vi "DWF FGEN Query Waveform Mode.vi"(0 "Instrument Handle In":u32, 11 "Error In":errorcluster caption="Error In (no error)") -> (4 "Instrument Handle Out":u32, 6 "Waveform Mode":i32(ring) items=["Standard", "Arbitrary"], 15 "Error Out":errorcluster)   [LabVIEW 2015, in "DigilentWF.lvlib"]
doc: "Indicates whether the waveform output by the instrument is a standard or arbitrary waveform."
uses:
  <vilib>/DigilentWF/DigilentWF.lvlib
  dwf.dll
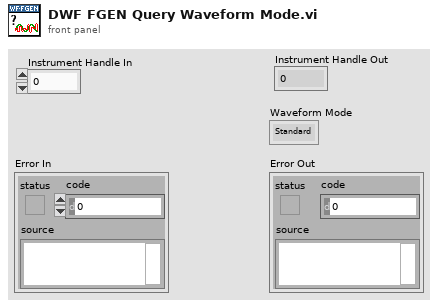
[diagram p1: front panel]
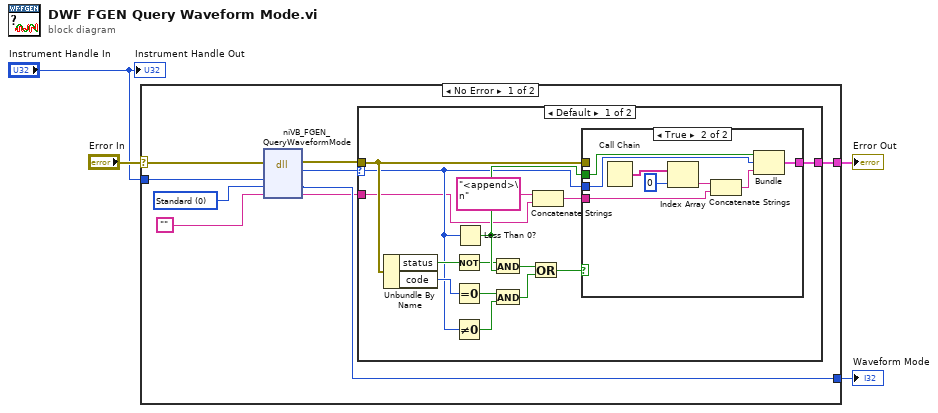
[diagram p0: block diagram]
diagram:
  n1 = case "outter_case" shown="No Error" "Error In" {
    selector: "Error In" -> [w12 w39]
    tunnel: [w13 w39] -> w3
    tunnel: "Instrument Handle In" -> [w10 _]
    tunnel: [w8 _] -> w1
    frame No Error {
      w9 = 0 items=["Standard", "Arbitrary"] ("Waveform Mode")
      n2 = dll-call lib="dwf.*" fn="niVB_FGEN_QueryWaveformMode"(error in=w12, "instrumentHandle"=w10, "waveformMode"=w9, "szError"="") -> (error out=w11:errorcluster, "return type"=w7:u32, "waveformMode"=w8:u32, "szError"=w5:string)  [unwired: 3 in, 1 out]
      n3 = case "inner_case" shown="Default" w7 {
        selector: w7 -> [w18 _]
        tunnel: w11 -> [w19 w38]
        tunnel: [w15 w38] -> w13
        tunnel: w5 -> [w14 _]
        frame Default {
          n4 = Unbundle By Name(w19) -> ("status"=w23:bool, "code"=w27:i32)
          n5 = Not(x=w23) -> (.not. x?=w26:bool)
          n6 = Equal To 0?(x=w27) -> (x = 0?=w22:bool)
          n7 = Not Equal To 0?(x=w18) -> (x != 0?=w25:bool)
          n8 = Less Than 0?(x=w18) -> (x < 0?=w28:bool)
          n9 = And(x=w26, y=w28) -> (x .and. y?=w24:bool)
          n10 = And(x=w22, y=w25) -> (x .and. y?=w21:bool)
          n11 = Or(x=w24, y=w21) -> (x .or. y?=w20:bool)
          n12 = Concatenate Strings("<append>\n" ("string"), w14) -> (w17:string)
          n13 = case shown="True" w20 {
            tunnel: [w29 w36] -> w15
            tunnel: w18 -> [_ w35]
            tunnel: w28 -> [_ w34]
            tunnel: w19 -> [w29 _]
            tunnel: w17 -> [_ w30]
            frame False {
            }
            frame True {
              n14 = Call Chain() -> (call chain=w33:string[])
              n15 = Index Array(array=w33, index=0) -> (element=w32:string)
              n16 = Concatenate Strings(w32, w30) -> (w37:string)
              n17 = Bundle(w34, "return type"=w35, w37) -> (w36:cluster{bool, "return type":u32, string})  [unwired: 1 out]
            }
          }
        }
        frame 0 {
        }
      }
    }
    frame Error {
    }
  }
  "Error Out" <- w3
  "Waveform Mode" <- w1
  "Instrument Handle Out" <- "Instrument Handle In"
